vi "pxie_7962_fpga.vi"() -> ()   [LabVIEW 2014]
uses:
  <instrlib>/_niInstr/Streaming/v1/Common/Stream State.ctl
  <vilib>/Platform/TimedLoop/XDataNode/timing_clust.ctl
  <vilib>/Platform/TimedLoop/XDataNode/nitl_modes.ctl
  <vilib>/Platform/TimedLoop/XDataNode/wakeup.ctl
  FPGA_Controls/Acquisition FIFOs Cluster.ctl
  <vilib>/rvi/Emulation/niFpgaSctlEmulationGetInTimedLoop.vi
  <vilib>/rvi/Emulation/niFpgaEmulationReportErrorSimple.vi
  <vilib>/rvi/Emulation/niFpgaGetClockAttributes.vi
  <vilib>/rvi/Emulation/niFpgaCriticalErrorInLSC.vi
  <vilib>/rvi/eio/common/nirviEmuTemplateMethod_errors.vi
  <instrlib>/_niInstr/Basic Elements/v1/FPGA/Private/D Latch U64.vi
  <vilib>/rvi/interface/RandomDataEmulation/niFpgaRandomDataHandleErrors.vi
  <vilib>/rvi/DataTransferAndStorage/Container/Common/niFpgaContainerExecOnDevCompGetState.vi
  <vilib>/rvi/Emulation/niFpgaEmulationIsFPGAContextNoSignature.vi
  <vilib>/rvi/errors/niFpgaSetErrorForExecOnDevCompSimple.vi
  <vilib>/rvi/eio/common/nirviEmuReportErrorAndStop.vi
  <vilib>/rvi/DataTransferAndStorage/Container/Common/niFpgaContainerGetUniqueNameForEmu.vi
  <vilib>/rvi/FIFO/Fifo_Resource/nirvififoEmulationSetSize.vi
  <vilib>/rvi/FIFO/Fifo_Resource/nirviFifoEmulationQueueMgr.vi
  <instcachedir>/0/nirviFifoEmulationQueueMgr_E5CAEC123FF24DC58D834DCA3CDAA9B5.lvgen/nirviFifoEmulationQueueMgr_E5CAEC123FF24DC58D834DCA3CDAA9B5_004.vi
  <vilib>/rvi/FIFO/Fifo_Resource/nirvififoEmulationDetermineInputValidOut.vi
  <vilib>/rvi/FIFO/Fifo_Resource/nirvififoEmulationCreateLock.vi
  <vilib>/rvi/Emulation/niFpgaProcessEmulError.vi
  <vilib>/rvi/FIFO/Fifo_Resource/nirvififoEmulationObtainLock.vi
  <vilib>/rvi/FIFO/Fifo_Resource/nirvififoEmulationReleaseLock.vi
  <vilib>/rvi/occurrence/nirviWaitOnOccurrenceBase.vi
  <vilib>/rvi/errors/nirviReportUnexpectedCaseInternalError.vi
  <vilib>/rvi/errors/nirviReportUnexpectedCaseInternalError (U32).vi
  <vilib>/Utility/error.llb/Clear Errors.vi
  <instcachedir>/0/nirviFifoEmulationQueueMgr_E5CAEC123FF24DC58D834DCA3CDAA9B5.lvgen/nirviFifoEmulationQueueMgr_E5CAEC123FF24DC58D834DCA3CDAA9B5_003.vi
  <vilib>/Platform/TimedLoop/XDataNode/XDataNode.xnode
  <vilib>/eio/EIONode/EIONode.xnode
  <vilib>/rvi/DataTransferAndStorage/Container/XNode/niFpgaContainer.xnode
  <vilib>/rvi/interface/RandomDataEmulation/nirviRandomDataFpgaReadWriteTemplate.vi
  <vilib>/rvi/FIFO/Fifo_Resource/niFpgaFifoEmulationRefIn.vi
  <vilib>/rvi/FIFO/Fifo_Resource/nirvififoEmulationWrite.vi
  <vilib>/Platform/TimedLoop/XDataNode/XDNodeRunTimeDep.lvlib
  <instrlib>/_niInstr/Streaming/v1/FPGA/niInstr Streaming v1 FPGA.lvlib
  <instrlib>/_niInstr/Basic Elements/v1/FPGA/niInstr Basic Elements v1 FPGA.lvlib
  <instrlib>/_niInstr/Streaming/v1/Common/niInstr Streaming v1 Common.lvlib
  <instrlib>/_niInstr/Basic Elements/v1/FPGA/Private/Count Up U64.vi
panel:
  out "Read Strobe before request":bool
  out "DRAM Init Done":bool
  in  "Reset DRAM read address":bool
  in  "Reset DRAM write address":bool
  in  "trigger \ncount":u64
  in  "Clear Trigger":bool
  in  "Debug":bool
  out "stream.metadata 0":u64
  in  "stream.request state 0":T1
  out "stream.samples transferred 0":u64
  out "stream.state 0":T1
  in  "stream.num samples 0":u64
  out "stream 1 \nidle state":bool
  out "stream 1 finite\ntransfer state":bool
  out "stream 1\ncancel state":bool
  out "stream 1\nnot ready state":bool
  out "stream 1\nerror state":bool
  out "Writes to DMA":u64
  out "Writes to \nDRAM":u64
  out "Writes to bundeling FIFO":u64
  out "Samples Aquired":u64
  out "IO Module Init Done":bool
  in  "stream.num samples 1":u64
  out "stream.state 1":T1
  out "stream.samples transferred 1":u64
  in  "stream.request state 1":T1
  out "stream.metadata 1":u64
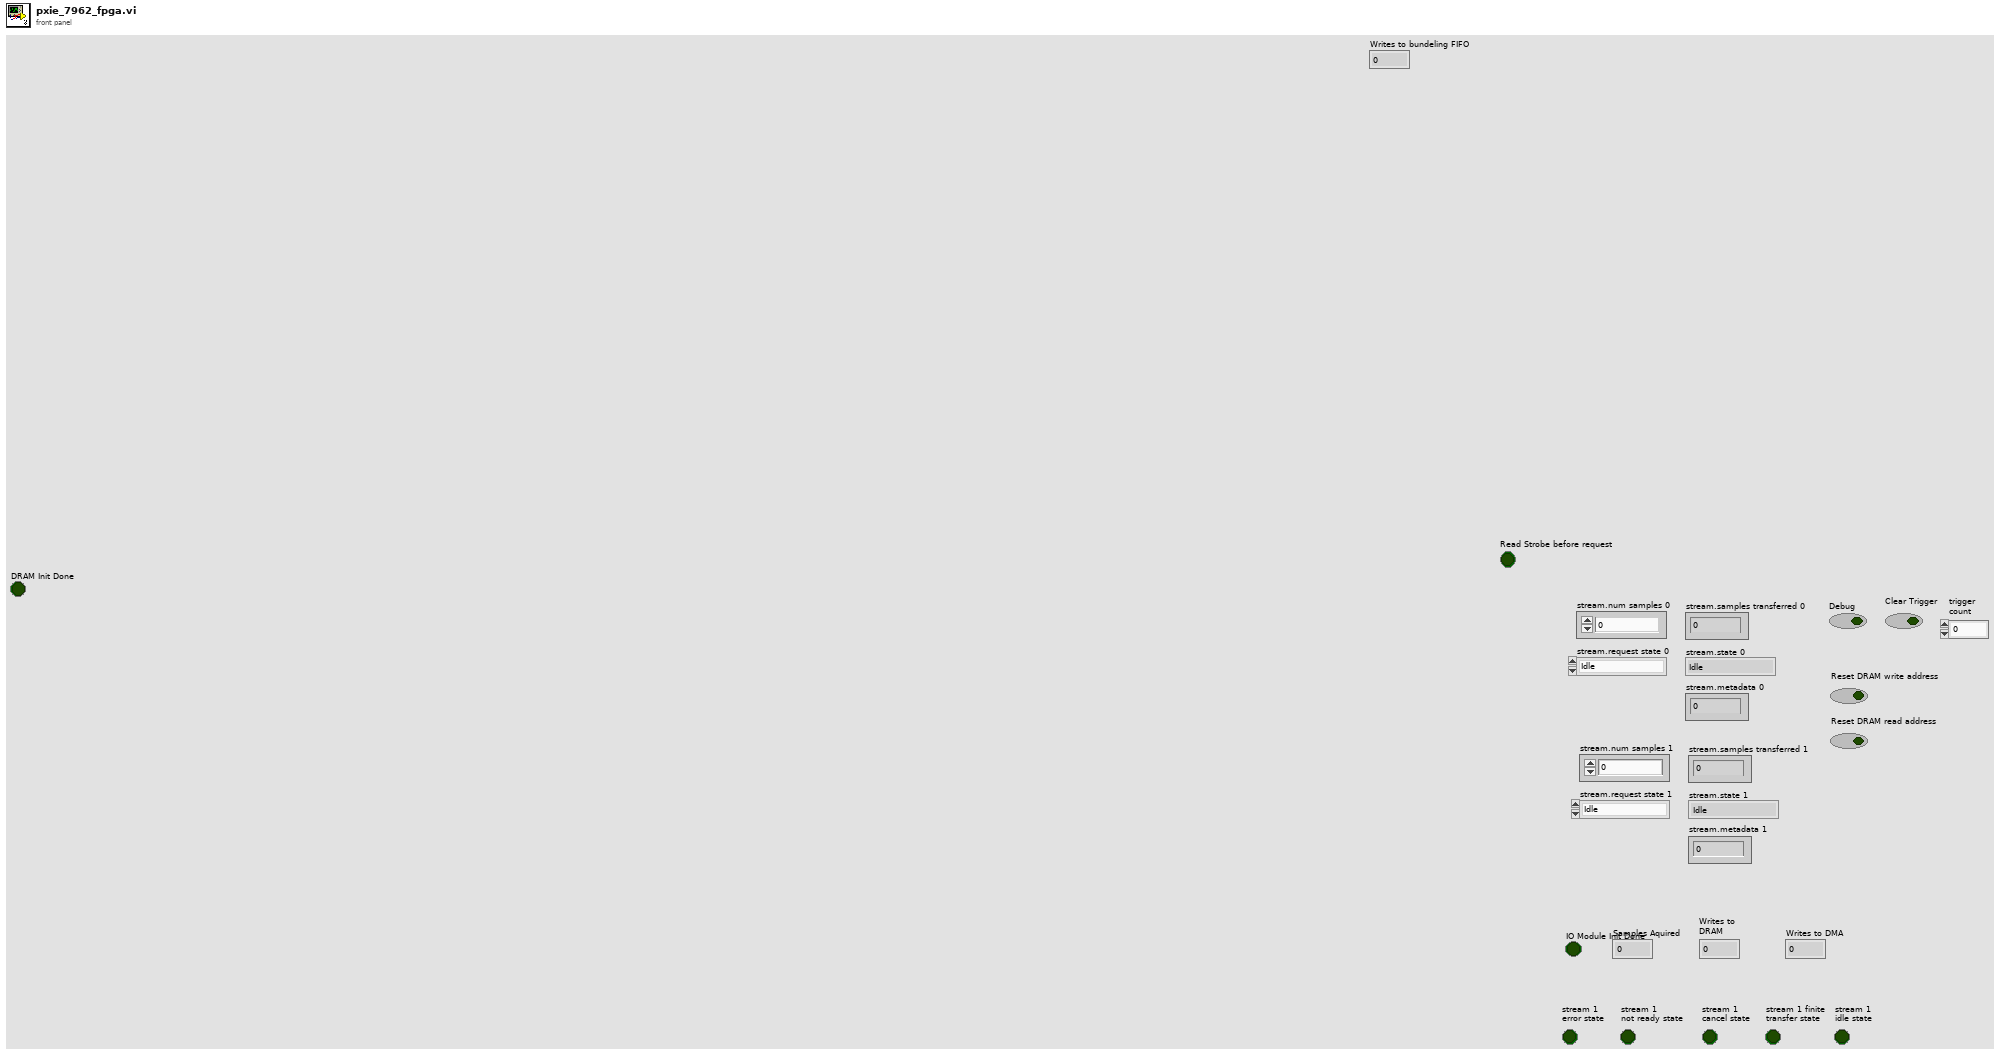
[diagram p1: front panel]
types:
  T1 = typedef "niInstr Streaming v1 Common.lvlib/Stream State.ctl" = enum8{"Idle", "Finite Transfer", "Continuous", "Done", "Error", "Not Ready", "Cancel"}
  T2 = typedef "XDNodeRunTimeDep.lvlib/timing_clust.ctl" = cluster{"Expected End [f-1]":u64, "Actual End [f-1]":u64, "Finished Late? [f-1]":bool, "Expected End [i-1]":u64, "Actual End [i-1]":u64, "Finished Late? [i-1]":bool, "Expected Start [i]":u64, "Actual Start [i]":u64, "Expected Start [f]":u64, "Actual Start [f]":u64, "Source Name":string, "Structure Name":string, "Period":i64, "Deadline":i64, "Offset":i64, "Start":i64, "Priority":i32, "Timeout":i32, "Mode":T3, "Wakeup Reason":T4, "Error":errorcluster, "Source Type":string, "Secondary Source Type":string, "Global End Time":u64, "Global Start Time":u64, "Frame Duration":u64, "Iteration Duration":u64, "Assigned CPU":i32, "I/O Scan Engine Mode":u32}
  T3 = typedef "XDNodeRunTimeDep.lvlib/nitl_modes.ctl" = enum32{"No Change", "Process missed periods, maintain original phase", "Discard missed periods, maintain original phase", "Process missed periods, ignore original phase", "Discard missed periods, ignore original phase"}
  T4 = typedef "XDNodeRunTimeDep.lvlib/wakeup.ctl" = enum32{"Normal", "Aborted", "Asynchronous wakeup", "Timing source error", "Timed loop error", "Timeout"}
  T5 = typedef "Acquisition FIFOs Cluster.ctl" = cluster{"FIFO 0":refnum<k21>, "FIFO 1":refnum<k21>, "FIFO 2":refnum<k21>, "FIFO 3":refnum<k21>, "FIFO 4":refnum<k21>, "FIFO 5":refnum<k21>, "FIFO 6":refnum<k21>, "FIFO 7":refnum<k21>}
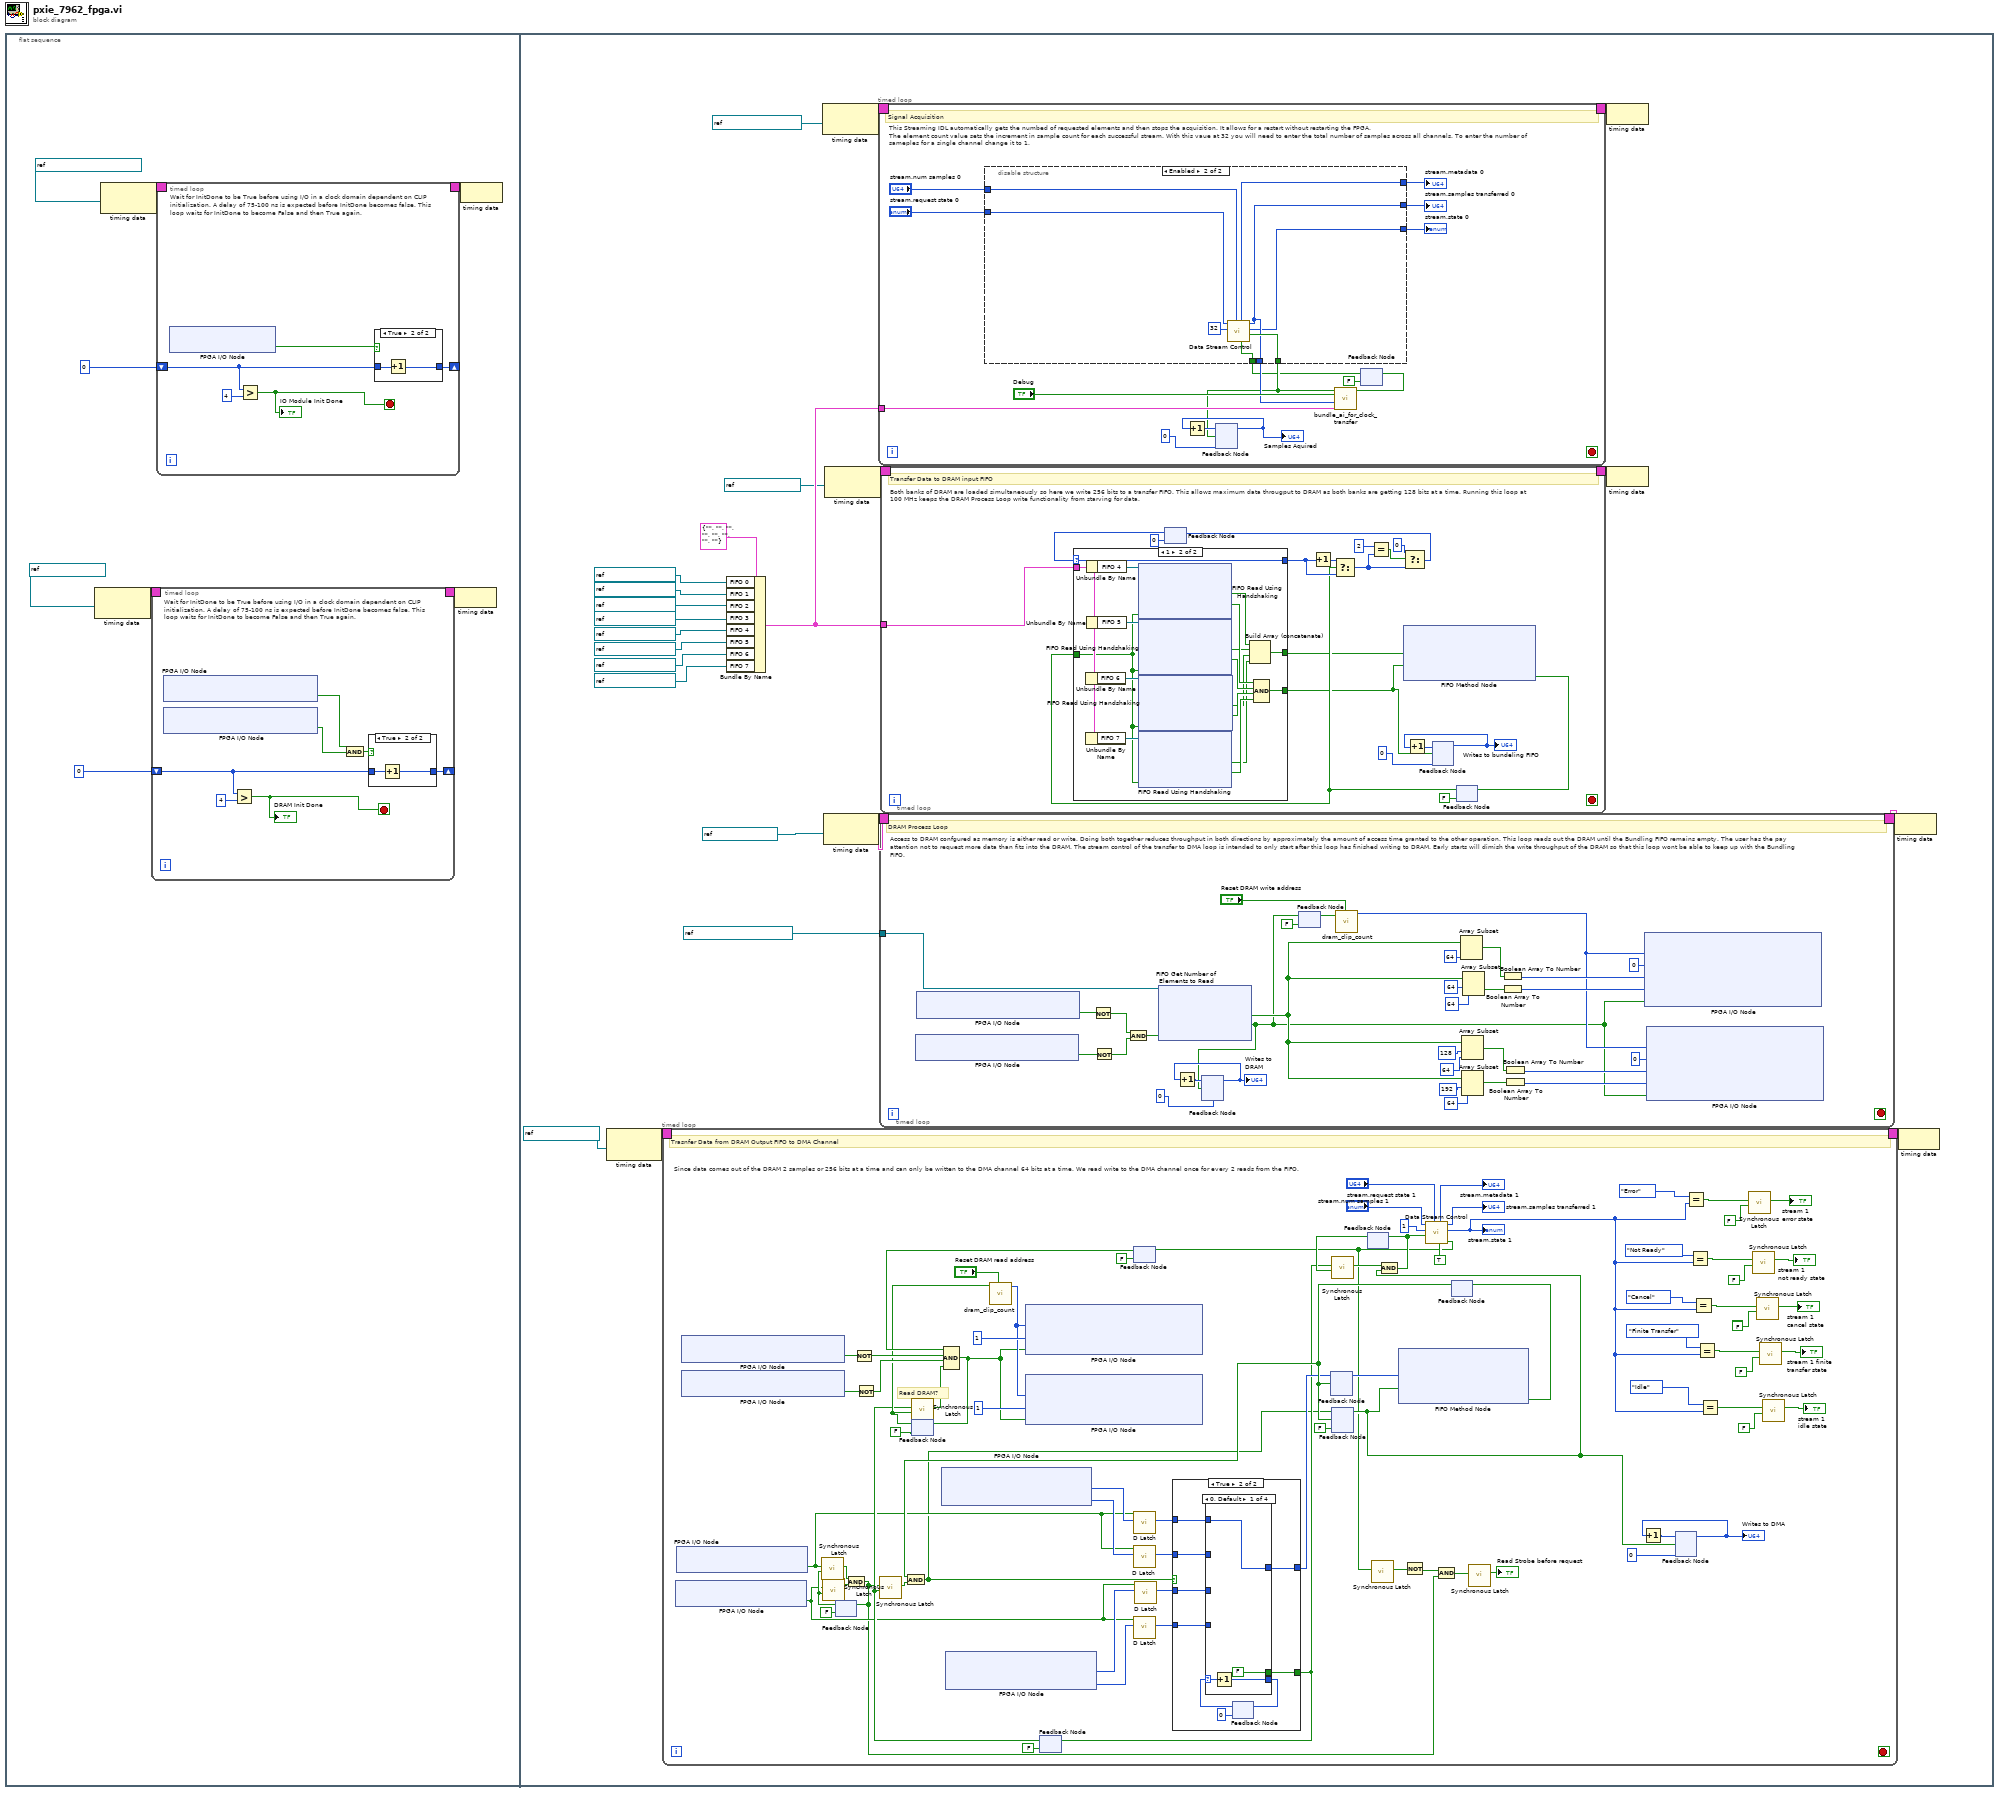
[diagram p0: block diagram]
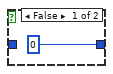
[diagram p2: hidden frame]
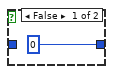
[diagram p3: hidden frame]
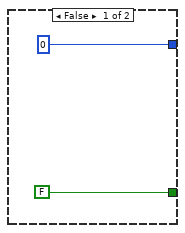
[diagram p4: hidden frame]
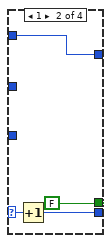
[diagram p5: hidden frame]
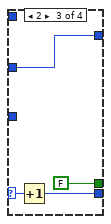
[diagram p6: hidden frame]
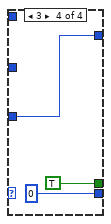
[diagram p7: hidden frame]
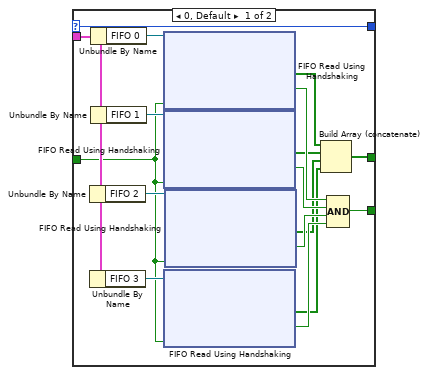
[diagram p8: hidden frame]
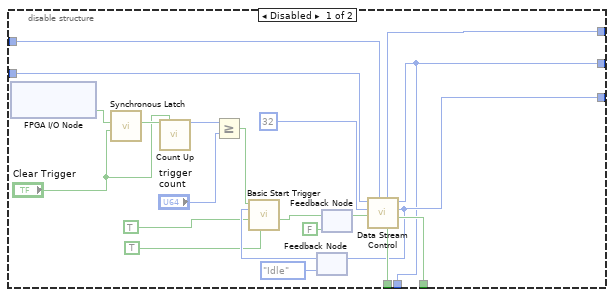
[diagram p9: hidden frame]
diagram:
  n1 = flat-sequence {
    frame #0 {
      n2 = node-c288(refnum<k21> "100 MHz Clock" ("Source Name")) -> (w4:T2)
      n3 = node-c288(refnum<k21> "40 MHz Onboard Clock" ("Source Name")) -> (w8:T2)
      n4 = timed-loop {
        shift-right: [w15] -> _
        shift-left: u16 0 -> [w14]
        timing: w4 -> [_]
        timing-out: [_] -> w3
        stop <- w12 stop-if-true
        # "Wait for InitDone to be True before using I/O in a clock domain dependent on CLIP initialization. A delay of 75-100 ns is expected before InitDone becomes false. This loop waits for InitDone to become False and then True again."
        n5 = xnode "FPGA I/O Node"() -> ("DRAM Bank 0\\Initialization_Done"=w10:bool)  [unwired: 1 in, 1 out]
        n6 = xnode "FPGA I/O Node"() -> ("DRAM Bank 1\\Initialization_Done"=w9:bool)  [unwired: 1 in, 1 out]
        n7 = Greater?(x=w14, y=u16 4) -> (0:w12:bool)
        "DRAM Init Done" <- w12
        n8 = And(x=w10, y=w9) -> (x .and. y?=w11:bool)
        n9 = case shown="True" w11 {
          tunnel: [u16 0 w18] -> w15
          tunnel: w14 -> [_ w17]
          frame False {
          }
          frame True {
            n10 = Increment(x=w17) -> (x+1=w18:u16)
          }
        }
      }
      n11 = timed-loop {
        shift-right: [w29] -> _
        shift-left: u16 0 -> [w28]
        timing: w8 -> [_]
        timing-out: [_] -> w7
        stop <- w26 stop-if-true
        # "Wait for InitDone to be True before using I/O in a clock domain dependent on CLIP initialization. A delay of 75-100 ns is expected before InitDone becomes false. This loop waits for InitDone to become False and then True again."
        n12 = xnode "FPGA I/O Node"() -> ("IO Module\\InitDone"=w25:bool)  [unwired: 1 in, 1 out]
        n13 = Greater?(x=w28, y=u16 4) -> (0:w26:bool)
        "IO Module Init Done" <- w26
        n14 = case shown="True" w25 {
          tunnel: [u16 0 w32] -> w29
          tunnel: w28 -> [_ w31]
          frame False {
          }
          frame True {
            n15 = Increment(x=w31) -> (x+1=w32:u16)
          }
        }
      }
      n16 = node-c288(w3) -> ()
      n17 = node-c288(w7) -> ()
    }
    frame #1 {
      n18 = node-c288(refnum<k21> "100 MHz Clock" ("Source Name")) -> (w55:T2)
      n19 = timed-loop {
        timing: w55 -> [_]
        timing-out: [_] -> w54
        stop <- _ stop-if-true
        (unwired) FALSE ("clear")
        # "Since data comes out of the DRAM 2 samples or 256 bits at a time and can only be written to the DMA channel 64 bits at a time. We read write to the DMA channel once for every 2 reads from the FIFO."
        # "Read DRAM?"
        # "Trasnfer Data from DRAM Output FIFO to DMA Channel"
        n20 = xnode "FPGA I/O Node"() -> ("DRAM Bank 1\\Read_Strobe"=w80:bool)  [unwired: 1 in, 1 out]
        n21 = xnode "FPGA I/O Node"() -> ("DRAM Bank 0\\Read_Strobe"=w81:bool)  [unwired: 1 in, 1 out]
        n22 = xnode "FPGA I/O Node"() -> ("DRAM Bank 0\\Command_FIFO_Full"=w109:bool)  [unwired: 1 in, 1 out]
        n23 = xnode "FPGA I/O Node"() -> ("DRAM Bank 1\\Command_FIFO_Full"=w110:bool)  [unwired: 1 in, 1 out]
        n24 = feedback #1(FALSE) -> (w99:bool)
        n25 = call <instrlib>:"Synchronous Latch.vi"("clear"=w99, "set"=w81) -> ("out"=w102:bool)  [unwired: 9 in]
        n26 = call <instrlib>:"Synchronous Latch.vi"("clear"=w99, "set"=w80) -> ("out"=w101:bool)  [unwired: 9 in]
        n27 = And(x=w102, y=w101) -> (x .and. y?=w64:bool)
        n28 = feedback-in #1(w64) -> ()
        n29 = Not(x=w109) -> (.not. x?=w106:bool)
        n30 = Not(x=w110) -> (.not. x?=w103:bool)
        n31 = feedback #2(FALSE ("set")) -> (w87:bool)
        n32 = xnode "FPGA I/O Node"() -> ("DRAM Bank 0\\Read_Data_Upper"=w85:u64, "DRAM Bank 0\\Read_Data_Lower"=w84:u64)  [unwired: 2 in, 2 out]
        n33 = xnode "FPGA I/O Node"() -> ("DRAM Bank 1\\Read_Data_Upper"=w83:u64, "DRAM Bank 1\\Read_Data_Lower"=w82:u64)  [unwired: 2 in, 2 out]
        n34 = call "dram_clip_count.vi"("reset"="Reset DRAM read address", "increment"=w87) -> ("count out"=w89:u32)  [unwired: 9 in]
        n35 = feedback #3(FALSE) -> (w86:bool)
        n36 = call <instrlib>:"Synchronous Latch.vi"("clear"=w86, "set"=w64) -> ("out"=w94:bool)  [unwired: 9 in]
        n37 = call <instrlib>:"Synchronous Latch.vi"("clear"=w87, "set"=w86) -> ("out"=w72:bool)  [unwired: 9 in]
        n38 = feedback #4(FALSE ("send data")) -> (w107:bool)
        n39 = Compound Arithmetic op=AND(w107, w106, w103, w72) -> (w71:bool)
        n40 = feedback-in #2(w71) -> ()
        n41 = xnode "FPGA I/O Node"("DRAM Bank 0\\Address"=w89, "DRAM Bank 0\\Command"=u8 1 ("DRAM Bank 0\\Command"), "DRAM Bank 0\\Command_Write_Enable"=w71) -> ()  [unwired: 3 in, 3 out]
        n42 = xnode "FPGA I/O Node"("DRAM Bank 1\\Address"=w89, "DRAM Bank 1\\Command"=u8 1 ("DRAM Bank 1\\Command"), "DRAM Bank 1\\Command_Write_Enable"=w71) -> ()  [unwired: 3 in, 3 out]
        n43 = call-poly <instrlib>:"D Latch.vi"("d"=w84, "s"=w81) -> ("q"=w78:u64)  [unwired: 9 in]
        n44 = call-poly <instrlib>:"D Latch.vi"("d"=w85, "s"=w81) -> ("q"=w79:u64)  [unwired: 9 in]
        n45 = call-poly <instrlib>:"D Latch.vi"("d"=w82, "s"=w80) -> ("q"=w76:u64)  [unwired: 9 in]
        n46 = call-poly <instrlib>:"D Latch.vi"("d"=w83, "s"=w80) -> ("q"=w77:u64)  [unwired: 9 in]
        n47 = feedback #5() -> (w70:u64)  [unwired: 1 in]
        n48 = feedback #6(FALSE ("out")) -> (w68:bool)
        n49 = feedback #7() -> (w90:bool)  [unwired: 1 in]
        n50 = xnode ("FIFO Method Node")("Element"=w70, "Input Valid"=w68) -> ("Ready for Input"=w69:bool)  [unwired: 1 in, 1 out]
        n51 = feedback-in #8(w69) -> ()
        n52 = feedback #8() -> (w93:bool)  [unwired: 1 in]
        n53 = And(x=w93, y=w94) -> (x .and. y?=w73:bool)
        n54 = case shown="True" w73 {
          tunnel: [u64 0 ("DRAM Bank 1\\Read_Data_Lower") w148] -> w75
          tunnel: [FALSE w147] -> w74
          tunnel: w79 -> [_ w146]
          tunnel: w78 -> [_ w145]
          tunnel: w77 -> [_ w144]
          tunnel: w76 -> [_ w143]
          frame False {
          }
          frame True {
            n55 = feedback #9(i16 0) -> (w150:i16)
            n56 = case shown="0, Default" w150 {
              selector: w150 -> [w154 w158 w162 _]
              tunnel: [w151 w155 w159 w163] -> w148
              tunnel: [w153 w157 w161 i16 0] -> w142
              tunnel: [FALSE FALSE FALSE TRUE] -> w147
              tunnel: w146 -> [w151 _ _ _]
              tunnel: w145 -> [_ w155 _ _]
              tunnel: w144 -> [_ _ w159 _]
              tunnel: w143 -> [_ _ _ w163]
              frame 0, Default {
                n57 = Increment(x=w154) -> (x+1=w153:i16)
              }
              frame 1 {
                n58 = Increment(x=w158) -> (x+1=w157:i16)
              }
              frame 2 {
                n59 = Increment(x=w162) -> (x+1=w161:i16)
              }
              frame 3 {
              }
            }
            n60 = feedback-in #9(w142) -> ()
          }
        }
        n61 = feedback-in #3(w74) -> ()
        n62 = feedback-in #5(w75, w93) -> ()
        n63 = call <instrlib>:"Synchronous Latch.vi"("clear"=w90, "set"=w74) -> ("out"=w92:bool)  [unwired: 9 in]
        n64 = feedback-in #6(w73, w93) -> ()
        n65 = And(x=w92, y=w68) -> (x .and. y?=w91:bool)
        n66 = feedback-in #7(w91) -> ()
        n67 = call <instrlib>:"Data Stream Control.vi"("ready for input?"=TRUE, "stream.num samples 0"="stream.num samples 1", "data valid"=w91, "element count"=u16 1, "stream.request state 0"="stream.request state 1") -> ("request data"=w67:bool, "stream.state 0"=w111:T1, "stream.samples transferred 0"=→"stream.samples transferred 1":u64, "stream.metadata 0"=→"stream.metadata 1":u64)  [unwired: 2 in, 1 out]
        "stream.state 1" <- w111
        n68 = feedback-in #4(w67) -> ()
        n69 = call <instrlib>:"Synchronous Latch.vi"("set"=w67) -> ("out"=w66:bool)  [unwired: 10 in]
        n70 = Not(x=w66) -> (.not. x?=w65:bool)
        n71 = And(x=w65, y=w64) -> (x .and. y?=w63:bool)
        n72 = call <instrlib>:"Synchronous Latch.vi"("set"=w63) -> ("out"=→"Read Strobe before request":bool)  [unwired: 10 in]
        n73 = feedback #10(u64 0) -> (w132:u64)
        "Writes to DMA" <- w132
        n74 = Increment(x=w132) -> (x+1=w133:u64)
        n75 = feedback-in #10(w133, w68) -> ()
        n76 = Equal?(x=Stream_State."Error" ("stream.state 0"), y=w111) -> (x = y?=w128:bool)
        n77 = Equal?(x=Stream_State."Not Ready" ("stream.state 0"), y=w111) -> (x = y?=w124:bool)
        n78 = Equal?(x=Stream_State."Cancel" ("stream.state 0"), y=w111) -> (x = y?=w120:bool)
        n79 = Equal?(x=Stream_State."Finite Transfer" ("stream.state 0"), y=w111) -> (x = y?=w116:bool)
        n80 = Equal?(x=Stream_State."Idle" ("stream.state 0"), y=w111) -> (x = y?=w113:bool)
        n81 = call <instrlib>:"Synchronous Latch.vi"("clear"=FALSE, "set"=w128) -> ("out"=→"stream 1\nerror state":bool)  [unwired: 9 in]
        n82 = call <instrlib>:"Synchronous Latch.vi"("clear"=FALSE, "set"=w124) -> ("out"=→"stream 1\nnot ready state":bool)  [unwired: 9 in]
        n83 = call <instrlib>:"Synchronous Latch.vi"("clear"=FALSE, "set"=w120) -> ("out"=→"stream 1\ncancel state":bool)  [unwired: 9 in]
        n84 = call <instrlib>:"Synchronous Latch.vi"("clear"=FALSE, "set"=w116) -> ("out"=→"stream 1 finite\ntransfer state":bool)  [unwired: 9 in]
        n85 = call <instrlib>:"Synchronous Latch.vi"("clear"=FALSE, "set"=w113) -> ("out"=→"stream 1 \nidle state":bool)  [unwired: 9 in]
      }
      n86 = Bundle By Name(cluster=T5 {"FIFO 0"="", "FIFO 1"="", "FIFO 2"="", "FIFO 3"="", "FIFO 4"="", "FIFO 5"="", "FIFO 6"="", "FIFO 7"=""} ("FIFO Refs"), "FIFO 0"=refnum<k21> "AI Bundle FIFO 0" ("FIFO In"), "FIFO 1"=refnum<k21> "AI Bundle FIFO 1" ("FIFO In"), "FIFO 2"=refnum<k21> "AI Bundle FIFO 2" ("FIFO In"), "FIFO 3"=refnum<k21> "AI Bundle FIFO 3" ("FIFO In"), "FIFO 4"=refnum<k21> "AI Bundle FIFO 4" ("FIFO In"), "FIFO 5"=refnum<k21> "AI Bundle FIFO 5" ("FIFO In"), "FIFO 6"=refnum<k21> "AI Bundle FIFO 6" ("FIFO In"), "FIFO 7"=refnum<k21> "AI Bundle FIFO 7" ("FIFO In")) -> (w43:T5)
      n87 = node-c288(refnum<k21> "IO Module Clock 0" ("Source Name")) -> (w61:T2)
      n88 = node-c288(refnum<k21> "100 MHz Clock" ("Source Name")) -> (w57:T2)
      n89 = node-c288(refnum<k21> "100 MHz Clock" ("Source Name")) -> (w59:T2)
      n90 = timed-loop {
        timing: w61 -> [_]
        timing-out: [_] -> w60
        tunnel: w43 -> [w277]
        stop <- _ stop-if-true
        # "This Streaming IDL automatically gets the numbed of requested elements and then stops the acquisition. It allows for a restart without restarting the FPGA. \nThe element count value sets the increment in sample count for each successful stream. With this vaue at 32 you will need to enter the total number of samples across all channels. To enter the number of sameples for a single channel change it to 1."
        # "Signal Acquisition"
        n91 = feedback #11(u64 0) -> (w278:u64)
        "Samples Aquired" <- w278
        n92 = Increment(x=w278) -> (x+1=w279:u64)
        n93 = feedback #12(FALSE ("Ready for Input")) -> (w273:bool)
        n94 = disable-structure shown="Enabled" {
          disable-tunnel: [w292 w307] -> w275
          disable-tunnel: [w302 w310] -> w274
          disable-tunnel: w273 -> [w294 w309]
          disable-tunnel: [w291 w308] -> w272
          disable-tunnel: [w292 w307] -> w271
          disable-tunnel: [w293 w306] -> w270
          disable-tunnel: "stream.num samples 0" -> [w289 w305]
          disable-tunnel: "stream.request state 0" -> [w290 w304]
          frame Disabled {
            n95 = xnode "FPGA I/O Node"() -> ("PXI_Star"=w288:bool)  [unwired: 1 in, 1 out]
            n96 = call <instrlib>:"Synchronous Latch.vi"("clear"="Clear Trigger", "set"=w288) -> ("out"=w287:bool)  [unwired: 9 in]
            n97 = call-poly <instrlib>:"Count Up.vi"("increment"=w287, "reset"="Clear Trigger") -> ("count out"=w286:u64)  [unwired: 13 in]
            n98 = Greater Or Equal?(x=w286, y="trigger \ncount") -> (x >= y?=w285:bool)
            n99 = feedback #13(Stream_State."Idle" ("stream.state 0")) -> (w301:T1)
            n100 = call <instrlib>:"Basic Start Trigger.vi"("ready for start trigger"=TRUE, "data valid?"=TRUE, "stream.state"=w301, "start trigger"=w285) -> ("data valid"=w297:bool)  [unwired: 7 in]
            n101 = feedback #14(FALSE ("data valid")) -> (w298:bool)
            n102 = feedback-in #14(w297) -> ()
            n103 = call <instrlib>:"Data Stream Control.vi"("ready for input?"=w294, "stream.num samples 0"=w289, "data valid"=w298, "element count"=u16 32, "stream.request state 0"=w290) -> ("send data"=w302:bool, "stream.state 0"=w293:T1, "stream.samples transferred 0"=w292:u64, "stream.metadata 0"=w291:u64)  [unwired: 2 in, 1 out]
            n104 = feedback-in #13(w293) -> ()
          }
          frame Enabled {
            n105 = call <instrlib>:"Data Stream Control.vi"("ready for input?"=w309, "stream.num samples 0"=w305, "element count"=u16 32, "stream.request state 0"=w304) -> ("send data"=w310:bool, "stream.state 0"=w306:T1, "stream.samples transferred 0"=w307:u64, "stream.metadata 0"=w308:u64)  [unwired: 3 in, 1 out]
          }
        }
        "stream.state 0" <- w270
        "stream.samples transferred 0" <- w271
        "stream.metadata 0" <- w272
        n106 = feedback-in #11(w279, w274) -> ()
        n107 = call "bundle_ai_for_clock_transfer.vi"("FIFO Refs"=w277, "sample"=w275, "Debug"="Debug", "Input Valid"=w274) -> ("Ready for Input"=w282:bool)  [unwired: 7 in]
        n108 = feedback-in #12(w282) -> ()
      }
      n109 = timed-loop {
        timing: w57 -> [_]
        timing-out: [_] -> w56
        tunnel: refnum<k21> "Bundling to DRAM FIFO" ("FIFO In") -> [w203]
        stop <- _ stop-if-true
        # "Access to DRAM confgured as memory is either read or write. Doing both together reduces throughput in both directions by approximately the amount of access time granted to the other operation. This loop reads out the DRAM until the Bundling FIFO remains empty. The user has the pay attention not to request more data than fits into the DRAM. The stream control of the transfer to DMA loop is intended to only start after this loop has finished writing to DRAM. Early starts will dimish the write throughput of the DRAM so that this loop wont be able to keep up with the Bundling FIFO."
        # "DRAM Process Loop"
        n110 = xnode "FPGA I/O Node"() -> ("DRAM Bank 1\\Command_FIFO_Full"=w182:bool)  [unwired: 1 in, 1 out]
        n111 = xnode "FPGA I/O Node"() -> ("DRAM Bank 0\\Command_FIFO_Full"=w180:bool)  [unwired: 1 in, 1 out]
        n112 = Not(x=w180) -> (.not. x?=w179:bool)
        n113 = Not(x=w182) -> (.not. x?=w181:bool)
        n114 = And(x=w179, y=w181) -> (x .and. y?=w183:bool)
        n115 = xnode ("FIFO Get Number of Elements to Read")("Ready for Output"=w183, "FIFO In"=w203) -> ("Element"=w194:bool[], "Output Valid"=w174:bool)  [unwired: 1 out]
        n116 = feedback #15(u64 0) -> (w189:u64)
        "Writes to \nDRAM" <- w189
        n117 = Increment(x=w189) -> (x+1=w190:u64)
        n118 = feedback-in #15(w190, w174) -> ()
        n119 = feedback #16(FALSE ("Output Valid")) -> (w173:bool)
        n120 = feedback-in #16(w174) -> ()
        n121 = call "dram_clip_count.vi"("reset"="Reset DRAM write address", "increment"=w173) -> ("count out"=w175:u32)  [unwired: 9 in]
        n122 = Array Subset(array=w194, length=64) -> (w198:bool[])  [unwired: 1 in]
        n123 = Array Subset(array=w194, index=128, length=64) -> (w191:bool[])
        n124 = Array Subset(array=w194, index=192, length=64) -> (w192:bool[])
        n125 = Array Subset(array=w194, index=64, length=64) -> (w199:bool[])
        n126 = Boolean Array To Number(Boolean array=w198) -> (number=w187:u64)
        n127 = Boolean Array To Number(Boolean array=w199) -> (number=w186:u64)
        n128 = Boolean Array To Number(Boolean array=w191) -> (number=w185:u64)
        n129 = Boolean Array To Number(Boolean array=w192) -> (number=w184:u64)
        n130 = xnode "FPGA I/O Node"("DRAM Bank 0\\Address"=w175, "DRAM Bank 0\\Command"=u8 0 ("DRAM Bank 0\\Command"), "DRAM Bank 0\\Write_Data_Upper"=w187, "DRAM Bank 0\\Write_Data_Lower"=w186, "DRAM Bank 0\\Command_Write_Enable"=w174) -> ()  [unwired: 5 in, 5 out]
        n131 = xnode "FPGA I/O Node"("DRAM Bank 1\\Address"=w175, "DRAM Bank 1\\Command"=u8 0 ("DRAM Bank 1\\Command"), "DRAM Bank 1\\Write_Data_Upper"=w185, "DRAM Bank 1\\Write_Data_Lower"=w184, "DRAM Bank 1\\Command_Write_Enable"=w174) -> ()  [unwired: 5 in, 5 out]
      }
      n132 = timed-loop {
        timing: w59 -> [_]
        timing-out: [_] -> w58
        tunnel: w43 -> [w227]
        stop <- _ stop-if-true
        # "Both banks of DRAM are loaded simultaneously so here we write 256 bits to a transfer FIFO. This allows maximum data througput to DRAM as both banks are getting 128 bits at a time. Running this loop at 100 MHz keeps the DRAM Process Loop write functionality from starving for data."
        # "Transfer Data to DRAM input FIFO"
        n133 = feedback #17(i16 0 ("t")) -> (w226:i16)
        n134 = feedback #18(u64 0) -> (w212:u64)
        "Writes to bundeling FIFO" <- w212
        n135 = Increment(x=w212) -> (x+1=w213:u64)
        n136 = feedback #19(FALSE ("Ready for Input")) -> (w215:bool)
        n137 = case shown="1" w226 {
          selector: w226 -> [w243 w260]
          tunnel: w227 -> [w229 w246]
          tunnel: [w241 w258] -> w210
          tunnel: [w234 w251] -> w211
          tunnel: [w243 w260] -> w223
          tunnel: w215 -> [w228 w245]
          frame 0, Default {
            n138 = Unbundle By Name(w229) -> ("FIFO 2"=w240:refnum<k21>)
            n139 = Unbundle By Name(w229) -> ("FIFO 3"=w239:refnum<k21>)
            n140 = Unbundle By Name(w229) -> ("FIFO 0"=w244:refnum<k21>)
            n141 = Unbundle By Name(w229) -> ("FIFO 1"=w242:refnum<k21>)
            n142 = xnode ("FIFO Read Using Handshaking")("Ready for Output"=w228, "FIFO In"=w244) -> ("Element"=w233:bool[], "Output Valid"=w238:bool)  [unwired: 1 out]
            n143 = xnode ("FIFO Read Using Handshaking")("Ready for Output"=w228, "FIFO In"=w242) -> ("Element"=w232:bool[], "Output Valid"=w237:bool)  [unwired: 1 out]
            n144 = xnode ("FIFO Read Using Handshaking")("Ready for Output"=w228, "FIFO In"=w239) -> ("Element"=w230:bool[], "Output Valid"=w235:bool)  [unwired: 1 out]
            n145 = xnode ("FIFO Read Using Handshaking")("Ready for Output"=w228, "FIFO In"=w240) -> ("Element"=w231:bool[], "Output Valid"=w236:bool)  [unwired: 1 out]
            n146 = Build Array (concatenate)(w233, w232, w231, w230) -> (w241:bool[])
            n147 = Compound Arithmetic op=AND(w238, w237, w236, w235) -> (w234:bool)
          }
          frame 1 {
            n148 = Unbundle By Name(w246) -> ("FIFO 6"=w257:refnum<k21>)
            n149 = Unbundle By Name(w246) -> ("FIFO 7"=w256:refnum<k21>)
            n150 = Unbundle By Name(w246) -> ("FIFO 4"=w261:refnum<k21>)
            n151 = Unbundle By Name(w246) -> ("FIFO 5"=w259:refnum<k21>)
            n152 = xnode ("FIFO Read Using Handshaking")("Ready for Output"=w245, "FIFO In"=w261) -> ("Element"=w250:bool[], "Output Valid"=w255:bool)  [unwired: 1 out]
            n153 = xnode ("FIFO Read Using Handshaking")("Ready for Output"=w245, "FIFO In"=w259) -> ("Element"=w249:bool[], "Output Valid"=w254:bool)  [unwired: 1 out]
            n154 = xnode ("FIFO Read Using Handshaking")("Ready for Output"=w245, "FIFO In"=w256) -> ("Element"=w247:bool[], "Output Valid"=w252:bool)  [unwired: 1 out]
            n155 = xnode ("FIFO Read Using Handshaking")("Ready for Output"=w245, "FIFO In"=w257) -> ("Element"=w248:bool[], "Output Valid"=w253:bool)  [unwired: 1 out]
            n156 = Build Array (concatenate)(w250, w249, w248, w247) -> (w258:bool[])
            n157 = Compound Arithmetic op=AND(w255, w254, w253, w252) -> (w251:bool)
          }
        }
        n158 = Increment(x=w223) -> (x+1=w224:i16)
        n159 = Select(t=w224, s=w215, f=w223) -> (s? t:f=w221:i16)
        n160 = Equal?(x=i16 2, y=w221) -> (x = y?=w220:bool)
        n161 = xnode ("FIFO Method Node")("Element"=w210, "Input Valid"=w211) -> ("Ready for Input"=w216:bool)  [unwired: 1 in, 1 out]
        n162 = Select(t=i16 0, s=w220, f=w221) -> (s? t:f=w219:i16)
        n163 = feedback-in #17(w219) -> ()
        n164 = feedback-in #18(w213, w211) -> ()
        n165 = feedback-in #19(w216) -> ()
      }
      n166 = node-c288(w60) -> ()
      n167 = node-c288(w58) -> ()
      n168 = node-c288(w56) -> ()
      n169 = node-c288(w54) -> ()
    }
  }
